vi "Create Dialog (by path).vi"(5 "Bar Visibility":T2={"Menu Bar"=FALSE, "Title Bar"=TRUE}, 6 "Calling VI Reference (caller)":refnum<vi>, 7 "Scrollbars (off)":T3, 8 "error in":errorcluster, 9 "Launch Position (Centered)":T1=enum."Centered", 10 "Dialog Behavior":T4(ring)=enum."Default", 11 "VI Path":path) -> (0 "error out":errorcluster, 3 "Flex Dialog out":refnum<class "Flex UI Dialog.lvclass">)   [LabVIEW 2016, in "Flex UI Dialog.lvclass"]
doc: "Generates a Dialog with all the associated behavior from the input UI VI Reference.\n\nIf no reference is given, uses the calling VI."
uses:
  Flex UI Dialog.lvclass
  Cluster - Scrollbar Settings.ctl
  Cluster - Bar Visibility.ctl
  Enum - Launch Position.ctl
  Flex UI (Parent)/Flex UI.lvclass
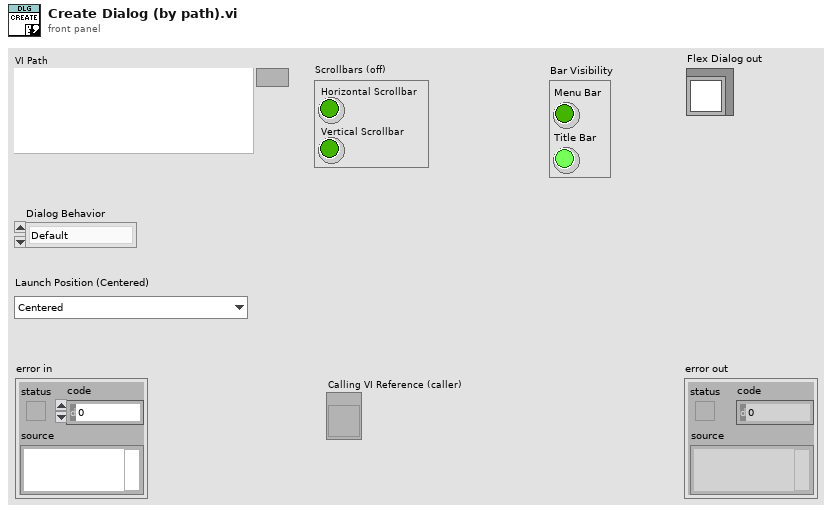
[diagram p1: front panel]
types:
  T1 = typedef "Flex UI Dialog.lvclass/Enum - Launch Position.ctl" = enum16{"Default (Last Opened)", "Centered", "Centered on Caller", "Maximized", "Hidden"}
  T2 = typedef "Flex UI Dialog.lvclass/Cluster - Bar Visibility.ctl" = cluster{"Menu Bar":bool, "Title Bar":bool}
  T3 = typedef "Flex UI Dialog.lvclass/Cluster - Scrollbar Settings.ctl" = cluster{"Horizontal Scrollbar":bool, "Vertical Scrollbar":bool}
  T4 = enum32{"Invalid", "Default", "Floating", "Floating/Auto-Hide", "Modal"}
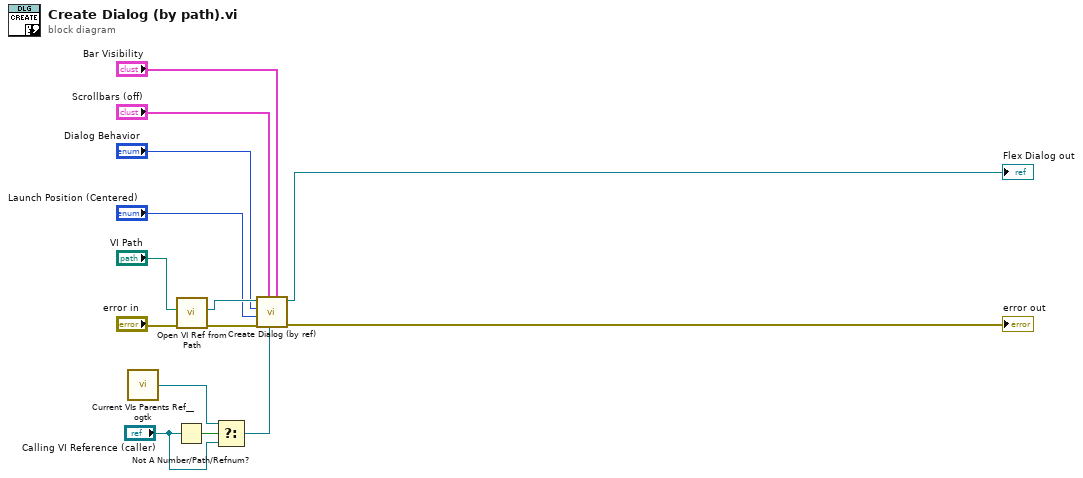
[diagram p0: block diagram]
diagram:
  n1 = call <userlib>:"Current VIs Parents Ref__ogtk.vi"() -> ("Calling VI's Reference"=w4:refnum<vi>)  [unwired: 2 in]
  n2 = Not A Number/Path/Refnum?(number/path/refnum="Calling VI Reference (caller)") -> (NaN/Path/Refnum?=w5:bool)
  n3 = call "Open VI Ref from Path.vi"("error in"="error in", "VI Path"="VI Path") -> ("error out"=w12:errorcluster, "VI Ref"=w10:refnum<vi>)  [unwired: 8 in]
  n4 = Select(t=w4, s=w5, f="Calling VI Reference (caller)") -> (s? t:f=w2:refnum<vi>)
  n5 = call "Create Dialog (by ref).vi"("Bar Visibility"="Bar Visibility", "Calling VI Reference"=w2, "Scrollbars (off)"="Scrollbars (off)", "error in"=w12, "Launch Position (Centered)"="Launch Position (Centered)", "Dialog Behavior"="Dialog Behavior", "UI VI Reference (caller)"=w10) -> ("error out"=→"error out":errorcluster, "Flex Dialog out"=→"Flex Dialog out":refnum<class "Flex UI Dialog.lvclass">)  [unwired: 3 in]
